vi "H5Gget_objtype_by_idx.vi"(6 "error in (no error)":errorcluster, 8 "Index":u64, 9 "HDF5 Ref":T2) -> (0 "error out":errorcluster, 2 "Object Type":T1 items=["H5G_UNKNOWN"=-1, "H5G_GROUP"=0, "H5G_DATASET"=1, "H5G_TYPE"=2, "H5G_LINK"=3, "H5G_UDLINK"=4], 3 "HDF5 Ref out":T2)   [LabVIEW 2017]
doc: "Returns the type of an object specified by an index."
uses:
  <vilib>/UPVI/lvhdf5/library.llb/HDF5 Ref.ctl
  <vilib>/UPVI/lvhdf5/group.llb/H5G_obj_t.ctl
  <vilib>/UPVI/lvhdf5/hdf5.dll
panel:
  # "LVHDF5 Toolkit\nCopyright (c) 2005-2013 by Jason D. Sommerville\nCopyright (c) 2014 by UPVI, LLC.\n\nThis use and distribution of this file is governed by the terms found in \nLICENSE.txt distributed with this toolkit and installed at\n <user.lib>\\_lvhdf5\\LICENSE.txt"
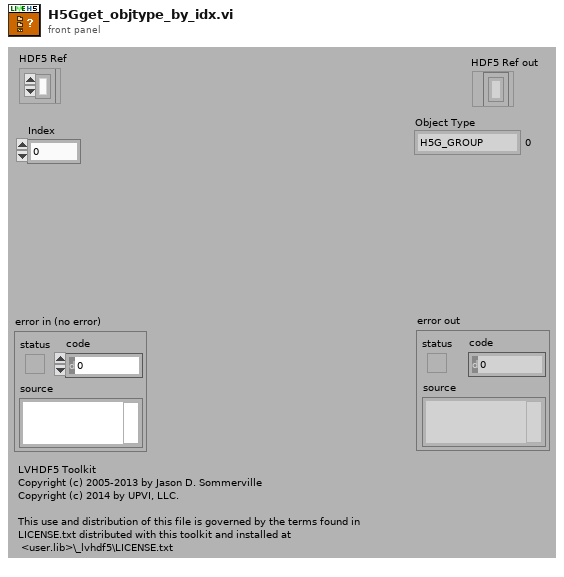
[diagram p1: front panel]
types:
  T1 = typedef "H5G_obj_t.ctl" = i32
  T2 = typedef "HDF5 Ref.ctl" = refnum<k1>
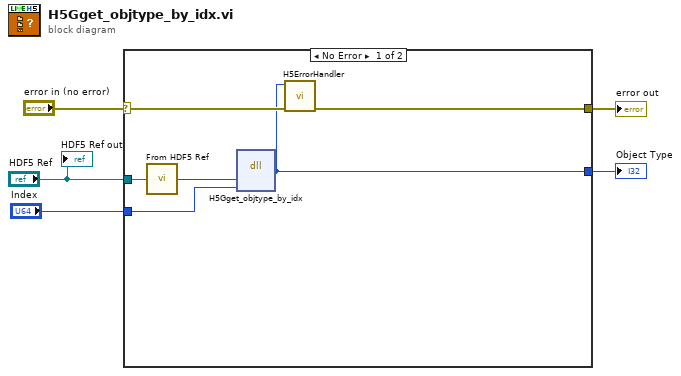
[diagram p0: block diagram]
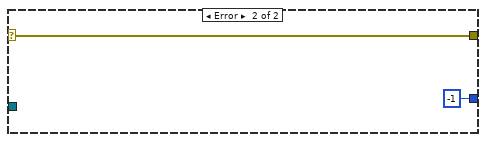
[diagram p2: hidden frame]
diagram:
  n1 = case shown="No Error" "error in (no error)" {
    selector: "error in (no error)" -> [w11 w13]
    tunnel: [w8 w13] -> w4
    tunnel: "HDF5 Ref" -> [w10 _]
    tunnel: "Index" -> [w6 _]
    tunnel: [w7 -1] -> w1
    frame No Error {
      n2 = call <vilib>:"From HDF5 Ref.vi"("HDF5 Ref"=w10) -> ("I32"=w9:i32)
      n3 = dll-call lib="C:/Program Files/National Instruments/LabVIEW 2017/vi.lib/UPVI/lvhdf5/hdf5.dll" fn="H5Gget_objtype_by_idx"("loc_id"=w9, "idx"=w6) -> ("return type"=w7:i32)  [unwired: 5 in, 2 out]
      n4 = call <vilib>:"H5ErrorHandler.vi"("error in (no error)"=w11, "herr_t"=w7) -> ("error out"=w8:errorcluster)  [unwired: 3 in, 4 out]
    }
    frame Error {
    }
  }
  "error out" <- w4
  "Object Type" <- w1
  "HDF5 Ref out" <- "HDF5 Ref"
